vi "RG Get Spectrum Wavelengths.vi"() -> (1 "Wavelength interval":i32, 2 "End wavelength":i32, 3 "Start wavelength":i32)   [LabVIEW 2017]
panel:
  in  "Wavelength interval":string="25"
  in  "End wavelength":string="800"
  in  "Cancel":bool
  in  "OK":bool
  in  "Start wavelength":string="500"
  # "Chose the wavelengths for your spectrum."
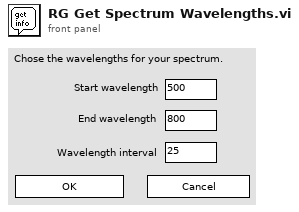
[diagram p1: front panel]
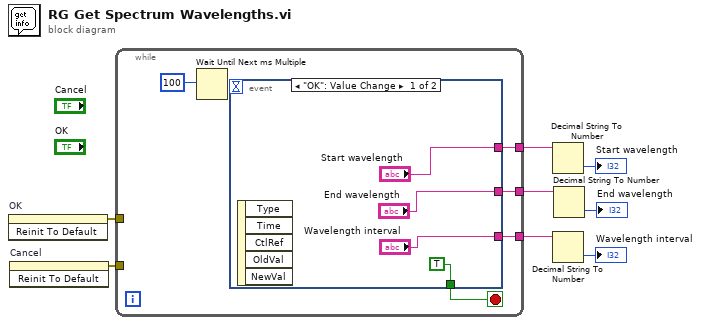
[diagram p0: block diagram]
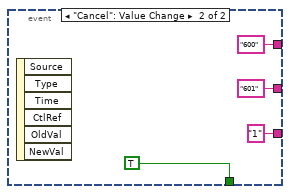
[diagram p2: hidden frame]
diagram:
  n1 = invoke on="OK" class="Bool" method="Reinit To Default"() -> (error out=w8:errorcluster)  [unwired: 3 in, 2 out]
  n2 = invoke on="Cancel" class="Bool" method="Reinit To Default"() -> (error out=w7:errorcluster)  [unwired: 3 in, 2 out]
  n3 = while {
    tunnel: [w13] -> w6
    tunnel: w8 -> [_]
    tunnel: w7 -> [_]
    tunnel: [w10] -> w2
    tunnel: [w9] -> w1
    stop <- w11 stop-if-true
    n4 = Wait Until Next ms Multiple(millisecond multiple=100) -> ()  [unwired: 1 out]
    n5 = event shown="[0] \"OK\": Value Change" {
      selector: _ -> [_ _]
      dyn-events: _ -> [_ _]
      timeout: _ -> [_ _]
      tunnel: [TRUE TRUE] -> w11
      tunnel: ["Start wavelength" "600" ("Start wavelength")] -> w13
      tunnel: ["End wavelength" "601" ("End wavelength")] -> w10
      tunnel: ["Wavelength interval" "1" ("Wavelength interval")] -> w9
      event "OK": Value Change {
        n6 = event-data() -> ()  [unwired: 6 out]
      }
      event "Cancel": Value Change {
        n7 = event-data() -> ()  [unwired: 7 out]
      }
    }
  }
  n8 = Decimal String To Number(string=w6) -> (number=→"Start wavelength":i32)  [unwired: 2 in, 1 out]
  n9 = Decimal String To Number(string=w1) -> (number=→"Wavelength interval":i32)  [unwired: 2 in, 1 out]
  n10 = Decimal String To Number(string=w2) -> (number=→"End wavelength":i32)  [unwired: 2 in, 1 out]
